vi "Init.vi"(8 "error in (no error)":errorcluster, 10 "CONTROLLER":refnum<class "CONTROLLER.lvclass">, 11 "VIEW in":refnum<class "VIEW.lvclass">) -> (0 "error out":errorcluster, 3 "VIEW out":refnum<class "VIEW.lvclass">)   [LabVIEW 2013, in "VIEW.lvclass"]
uses:
  VIEW.lvclass
  Controller/base/CONTROLLER.lvclass
  VIEW.lvclass/VIEW.ctl
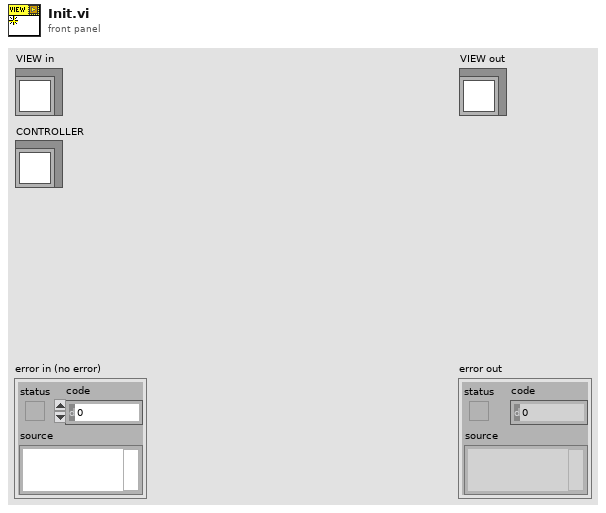
[diagram p1: front panel]
types:
  T1 = cluster{"CtlRef":refnum<vi>, "Name":string, "ClassName":string}
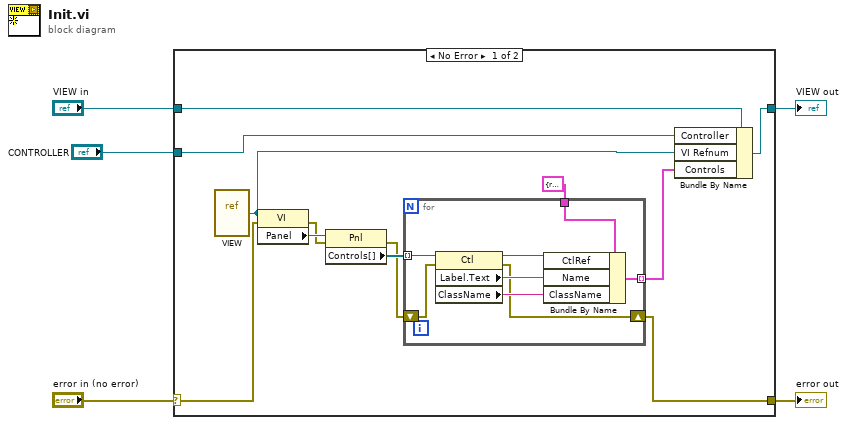
[diagram p0: block diagram]
diagram:
  n1 = case shown="No Error" "error in (no error)" {
    selector: "error in (no error)" -> [w11 w27]
    tunnel: [w10 w27] -> w4
    tunnel: [w8 w26] -> w2
    tunnel: "VIEW in" -> [w9 w26]
    tunnel: "CONTROLLER" -> [w6 _]
    frame No Error {
      n2 = vi-ref "VIEW.vi"() -> (w7:refnum<vi>)
      n3 = property class="VI"(reference=w7, error in=w11) -> (error out=w16:errorcluster, "Panel"=w17:refnum<vi>)  [unwired: 1 out]
      n4 = property class="Pnl"(reference=w17, error in=w16) -> (error out=w12:errorcluster, "Controls[]"=w15:refnum<vi>[])  [unwired: 1 out]
      n5 = for {
        tunnel: w15 -> [w25] mode=indexing
        tunnel: T1 {"CtlRef"=refnum, "Name"="", "ClassName"=""} ("CtlInfo") -> [w24]
        tunnel: [w20] -> w13 mode=indexing
        shift-right: [w18] -> w10
        shift-left: w12 -> [w19]
        n6 = property class="Ctl"(reference=w25, error in=w19) -> (reference out=w23:refnum<vi>, error out=w18:errorcluster, "Label.Text"=w22:string, "ClassName"=w21:string)
        n7 = Bundle By Name(cluster=w24, "CtlRef"=w23, "Name"=w22, "ClassName"=w21) -> (w20:T1)
      }
      n8 = Bundle By Name(cluster=w9, "Controller"=w6, "VI Refnum"=w7, "Controls"=w13) -> (w8:refnum<class "VIEW.lvclass">)
    }
    frame Error {
    }
  }
  "error out" <- w4
  "VIEW out" <- w2
